vi "hse-application_SystemConfiguration_ValidateUnit.vi"(8 "error in (no error)":errorcluster, 11 "hse-application in":refnum<class "hse-application.lvclass">) -> (0 "error out":errorcluster, 3 "hse-application DUP":refnum<class "hse-application.lvclass">)   [LabVIEW 2020, in "hse-application.lvclass"]
doc: "Check if <b>Unit Directory</b> exists. \n\n____\nHAMPEL SOFTWARE ENGINEERING v3.8.0 (2023-12-18 14:41)"
uses:
  hse-application.lvclass
  hse-application.lvclass/hse-application.ctl
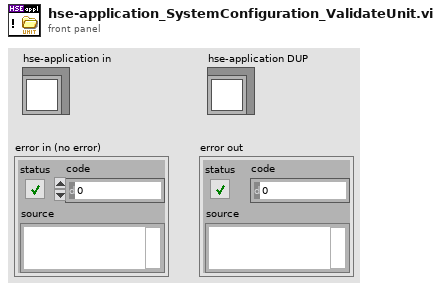
[diagram p1: front panel]
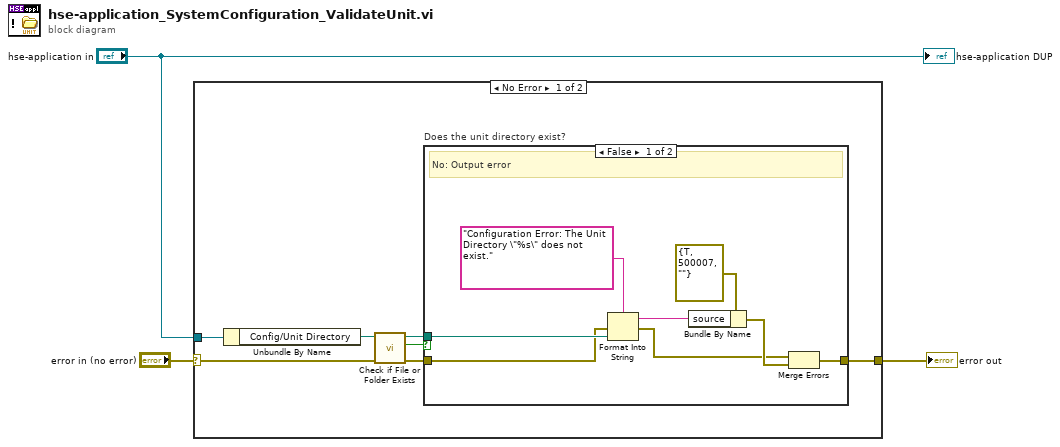
[diagram p0: block diagram]
diagram:
  n1 = case shown="No Error" "error in (no error)" {
    selector: "error in (no error)" -> [w10 w20]
    tunnel: [w7 w20] -> w3
    tunnel: "hse-application in" -> [w5 _]
    frame No Error {
      n2 = Unbundle By Name(w5) -> ("Config/Unit Directory"=w4:path)
      n3 = call <vilib>:"Check if File or Folder Exists.vi"("error in (no error)"=w10, "path"=w4) -> ("error out"=w8:errorcluster, "file or folder exists?"=w9:bool, "dup path"=w6:path)  [unwired: 7 in]
      n4 = case "Does the unit directory exist?" shown="False" w9 {
        tunnel: w8 -> [w13 w19]
        tunnel: [w12 w19] -> w7
        tunnel: w6 -> [w14 _]
        frame False {
          # "No: Output error"
          n5 = Format Into String(format string="Configuration Error: The Unit Directory \"%s\" does not exist.", error in=w13, w14) -> (resulting string=w16:string, error out=w11:errorcluster)  [unwired: 1 in]
          n6 = Bundle By Name(cluster=errorcluster {"status"=TRUE, "code"=500007, "source"=""} ("error out"), "source"=w16) -> (w18:errorcluster)
          n7 = Merge Errors(w11, w18) -> (w12:errorcluster)
        }
        frame True {
          # "Yes: Do nothing."
        }
      }
    }
    frame Error {
    }
  }
  "error out" <- w3
  "hse-application DUP" <- "hse-application in"
